vi "sub_applyGuess.vi"(9 "list of guesses":T1[](array[typedef]), 11 "solver (in)":T2[][](array[typedef])) -> (3 "solver (out)":T2[][](array[typedef]))   [LabVIEW 2018]
uses:
  cell.ctl
  guess.ctl
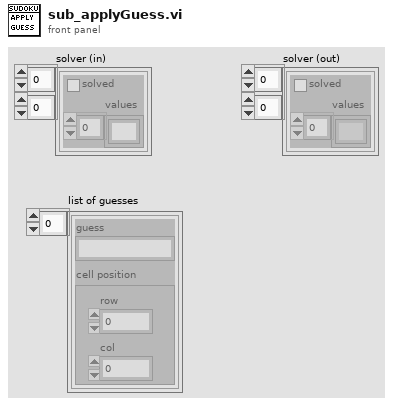
[diagram p1: front panel]
types:
  T1 = typedef "guess.ctl" = cluster{"cell position":cluster{"row":i32, "col":i32}, "guess":string}
  T2 = typedef "cell.ctl" = cluster{"solved":bool, "values":string[]}
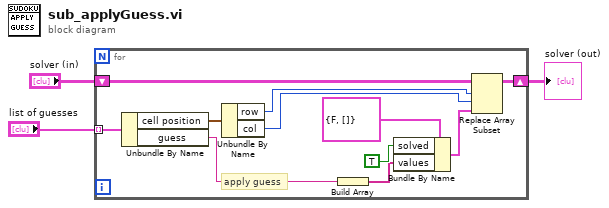
[diagram p0: block diagram]
diagram:
  n1 = for {
    shift-right: [w10] -> w1
    shift-left: "solver (in)" -> [w4]
    tunnel: "list of guesses" -> [w9] mode=indexing
    # "apply guess"
    n2 = Unbundle By Name(w9) -> ("cell position"=w8:cluster{"row":i32, "col":i32}, "guess"=w14:string)
    n3 = Unbundle By Name(w8) -> ("row"=w6:i32, "col"=w5:i32)
    n4 = Build Array(w14) -> (w7:string[])
    n5 = Bundle By Name(cluster=T2 {"solved"=FALSE, "values"=[]} ("cell"), "solved"=TRUE, "values"=w7) -> (w11:T2)
    n6 = Replace Array Subset(array=w4, new element=w11, index (row)=w6, index (col)=w5) -> (w10:T2[][])
  }
  "solver (out)" <- w1
